vi "Set Visibility.vi"(8 "error in (no error)":errorcluster, 10 "Visible":bool, 11 "Panel in":refnum<class "Panel.lvclass">) -> (0 "error out":errorcluster, 3 "Panel out":refnum<class "Panel.lvclass">)   [LabVIEW 2018]
uses:
  Panel Visibility Changed.ctl
  Panel.lvclass
  State.ctl
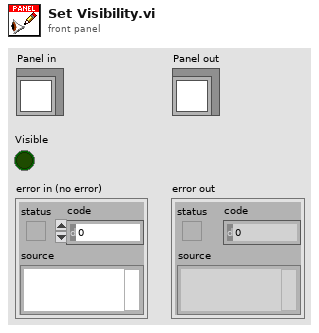
[diagram p1: front panel]
types:
  T1 = typedef "OOPanel.lvlib/Panel.lvclass/Panel Visibility Changed.ctl" = cluster{"State":T2}
  T2 = typedef "OOPanel.lvlib/Panel.lvclass/State.ctl" = enum16{"Idle", "Hidden", "Visible", "Subpanel"}
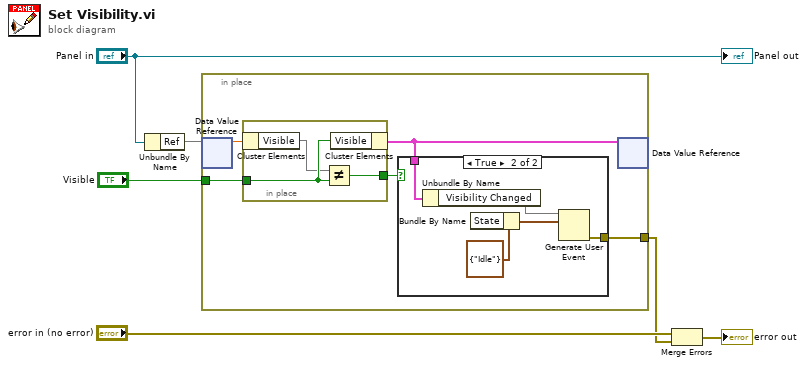
[diagram p0: block diagram]
diagram:
  n1 = Unbundle By Name("Panel in") -> ("Ref"=w4)
  n2 = in-place {
    in-place-border: "Visible" -> [w8]
    in-place-border: [w7] -> w1
    n3 = in-place-dvr #1(w4) -> (w11:dbl)  [unwired: 1 out]
    n4 = in-place {
      in-place-border: w8 -> [w19]
      in-place-border: [w17] -> w10
      n5 = in-place-cluster #2(w11) -> ("Visible"=w18)
      n6 = Not Equal?(x=w18, y=w19) -> (x != y?=w17:bool)
      n7 = in-place-cluster #2("Visible"=w19) -> (w9:cluster{})
    }
    n8 = case shown="True" w10 {
      tunnel: w9 -> [_ w16]
      tunnel: [_ w12] -> w7
      frame False {
      }
      frame True {
        n9 = Unbundle By Name(w16) -> ("Visibility Changed"=w15)
        n10 = Bundle By Name(cluster=T1 {"State"=enum."Idle"} ("Panel Visibility Changed")) -> (w13:T1)  [unwired: 1 in]
        n11 = Generate User Event(user event=w15, event data cluster=w13) -> (error out=w12:errorcluster)  [unwired: 2 in, 1 out]
      }
    }
    n12 = in-place-dvr #1(w9) -> ()  [unwired: 2 out]
  }
  n13 = Merge Errors("error in (no error)", w1) -> (→"error out":errorcluster)
  "Panel out" <- "Panel in"
